vi "gfitsio-get-column-number.vi"(6 "case sensitive? (F:No)":bool, 7 "column":string, 8 "error in (no error)":errorcluster, 11 "gfits refnum":T1) -> (0 "error out":errorcluster, 2 "colnum":i32, 3 "dup gfits refnum":T1)   [LabVIEW 2019, in "gfitsio.lvlib"]
doc: "Get the table column number of the column whose name matches an input template name. As a general rule, the column names should be treated as case INsensitive.\n\nThe input column name template may be either the exact name of the column to be searched for, or it may contain wild card characters (*, ?, or #), or it may contain the integer number of the desired column (with the first column = 1). The `*' wild card character matches any sequence of characters (including zero characters) and the `?' character matches any single character. The # wildcard will match any consecutive string of decimal digits (0-9). If more than one column name in the table matches the template string, then the first match is returned.\n\nThe FITS Standard recommends that only letters, digits, and the underscore character be used in column names (with no embedded spaces). Trailing blank characters are not significant. It is recommended that all the column names in a given table be unique within the first 8 characters, and strongly recommended that the names be unique within the first 16 characters."
uses:
  gfitsio.lvlib
  gfitsio-refnum.ctl
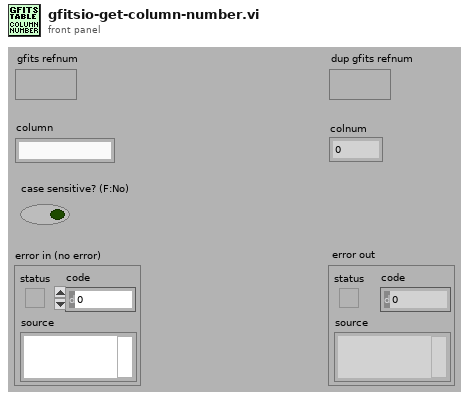
[diagram p1: front panel]
types:
  T1 = typedef "gfitsio.lvlib/gfitsio-refnum.ctl" = refnum<k1>
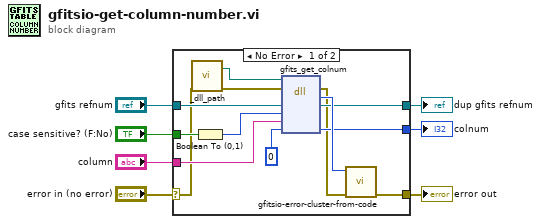
[diagram p0: block diagram]
diagram:
  n1 = case shown="No Error" "error in (no error)" {
    selector: "error in (no error)" -> [w10 w21]
    tunnel: [w18 w21] -> w7
    tunnel: "gfits refnum" -> [w16 w20]
    tunnel: [w17 w20] -> w5
    tunnel: [w11 _] -> w3
    tunnel: "column" -> [w13 _]
    tunnel: "case sensitive? (F:No)" -> [w15 _]
    frame No Error {
      n2 = call "_dll_path.vi"() -> ("Path"=w8:path)  [unwired: 1 in]
      n3 = Boolean To (0,1)(Boolean=w15) -> (0, 1=w14:i16)
      n4 = dll-call lib="?" fn="gfits_get_colnum"(path in=w8, error in=w10, "refnum"=w16, "casesen"=w14, "column"=w13, "colnum"=0) -> (error out=w9:errorcluster, "return type"=w19:i32, "refnum"=w17:T1, "colnum"=w11:i32)  [unwired: 2 in, 2 out]
      n5 = call "gfitsio-error-cluster-from-code.vi"("error in (no error)"=w9, "error code"=w19) -> ("error out"=w18:errorcluster)  [unwired: 9 out]
    }
    frame Error {
    }
  }
  "error out" <- w7
  "dup gfits refnum" <- w5
  "colnum" <- w3
